vi "TestAcq_NextStep.vi"(8 "error in":errorcluster, 10 "TestData":T1={"FilesPath"=path "", "Name_Meas"="", "stop"=FALSE, "Command"=enum."Start", "Fs"=1000.0, "Test"=FALSE}, 11 "Previous Step":T3) -> (0 "error out":errorcluster, 3 "Next Step":T3)   [LabVIEW 2019]
uses:
  TypeDef/#TypeDef_StateAcq.ctl
  TypeDef/#TypeDef_DataToTest.ctl
  Communication/TypeDef/#TypeDef_Command.ctl
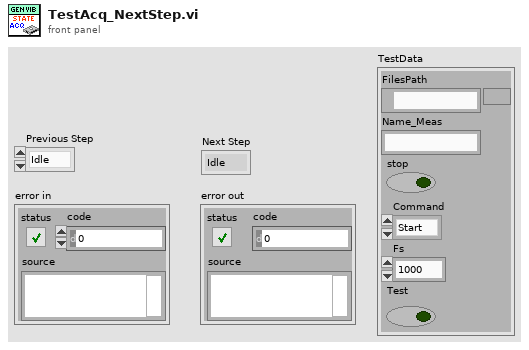
[diagram p1: front panel]
types:
  T1 = typedef "#TypeDef_DataToTest.ctl" = cluster{"FilesPath":path, "Name_Meas":string, "stop":bool, "Command":T2, "Fs":dbl, "Test":bool}
  T2 = typedef "#TypeDef_Command.ctl" = enum16{"Start", "End"}
  T3 = typedef "#TypeDef_StateAcq.ctl" = enum16{"Idle", "Init", "Acq", "End"}
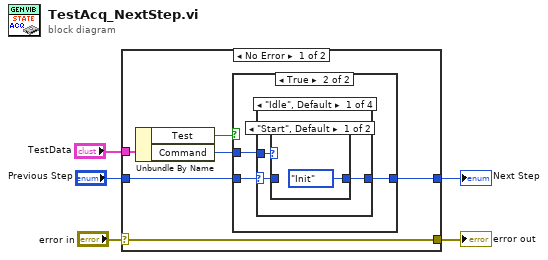
[diagram p0: block diagram]
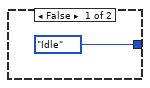
[diagram p2: hidden frame]
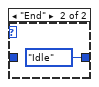
[diagram p3: hidden frame]
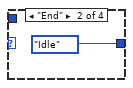
[diagram p4: hidden frame]
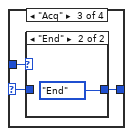
[diagram p5: hidden frame]
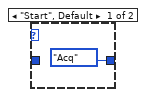
[diagram p6: hidden frame]
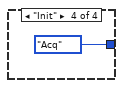
[diagram p7: hidden frame]
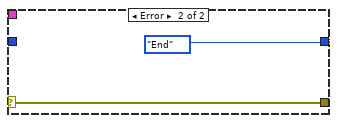
[diagram p8: hidden frame]
diagram:
  n1 = case shown="No Error" "error in" {
    selector: "error in" -> [w11 w29]
    tunnel: [w11 w29] -> w2
    tunnel: [w9 #TypeDef_StateAcq."End"] -> w5
    tunnel: "Previous Step" -> [w10 _]
    tunnel: "TestData" -> [w8 _]
    frame No Error {
      n2 = Unbundle By Name(w8) -> ("Test"=w6:bool, "Command"=w7:T2)
      n3 = case shown="True" w6 {
        tunnel: w10 -> [_ w15]
        tunnel: [#TypeDef_StateAcq."Idle" w14] -> w9
        tunnel: w7 -> [_ w13]
        frame False {
        }
        frame True {
          n4 = case shown="\"Idle\", Default" w15 {
            selector: w15 -> [w17 _ w23 _]
            tunnel: w13 -> [w18 _ w22 _]
            tunnel: [w16 #TypeDef_StateAcq."Idle" w24 #TypeDef_StateAcq."Acq"] -> w14
            frame "Idle", Default {
              n5 = case shown="\"Start\", Default" w18 {
                tunnel: [#TypeDef_StateAcq."Init" #TypeDef_StateAcq."Idle"] -> w16
                tunnel: w17 -> [_ _]
                frame "Start", Default {
                }
                frame "End" {
                }
              }
            }
            frame "End" {
            }
            frame "Acq" {
              n6 = case shown="\"End\"" w22 {
                tunnel: [#TypeDef_StateAcq."Acq" #TypeDef_StateAcq."End"] -> w24
                tunnel: w23 -> [_ _]
                frame "Start", Default {
                }
                frame "End" {
                }
              }
            }
            frame "Init" {
            }
          }
        }
      }
    }
    frame Error {
    }
  }
  "error out" <- w2
  "Next Step" <- w5
